vi "thermometric_station.vi"() -> ()   [LabVIEW 2017]
uses:
  dd87deb7-d795-4f28-a263-11bfb0a382d3.vi
  <vilib>/MakerHub/LINX/Public/Utilities/Open Serial.vi
  <vilib>/Utility/file.llb/Write Delimited Spreadsheet (string).vi
  <vilib>/MakerHub/LINX/LMH-LINX.lvlib
panel:
  in  "Stop":bool
  in  "Tab Control":T1(tab)
  out "Value Change":bool
  in  "Acquisition time":string(combo)
  in  "Save Button":bool
  out "Temperature (C)":u8(knob) scale=0.0..50.0
  out "Humidity (%)":u8(knob) scale=0.0..100.0
  in  "Serial Port":refnum<visa-resource-name>="N/A"
  out "Humidity":u8(graph)=43
  out "Temperature":u8(graph)
  out "HTML Content":string
  out "Cleaned Content":string
  out "Error Out":errorcluster
  out "Data":string[](array[string])
  in  "Table":string(combo)
  in  "Connection Information":path
  in  "Columns":string[](array[string])
  in  "Condition":string(combo)
  out "DB read":string[][](array[string])
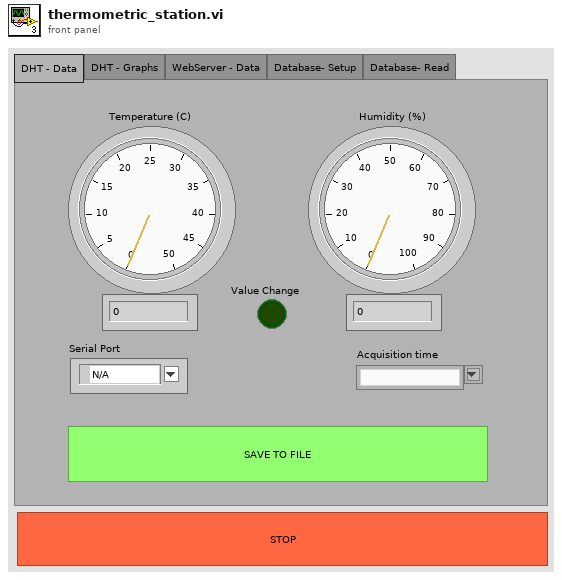
[diagram p1: front panel]
types:
  T1 = enum32{"DHT - Data", "DHT - Graphs", "WebServer - Data", "Database- Setup", "Database- Read"}
  T2 = typedef "LMH-LINX.lvlib/LINX Ref.ctl" = cluster{"IO":T3, "Interface":T4, "LINX Device Config":T5}
  T3 = typedef "LMH-LINX.lvlib/Platform.ctl" = enum16{"Remote", "Local"}
  T4 = typedef "LMH-LINX.lvlib/Interface.ctl" = enum16{"Serial", "TCP"}
  T5 = typedef "LMH-LINX.lvlib/Device.lvlib/LINX Device Config.ctl" = cluster{"Interface":T4, "COM Port":refnum<visa-resource-name>, "TCP Configuration":T6, "Device Family":u8, "Device ID":u8, "Device Name":string, "TCP Ref":refnum<k5>, "Channels":T7}
  T6 = typedef "LMH-LINX.lvlib/Device.lvlib/TCP Config.ctl" = cluster{"IP Address":string, "Port":u16}
  T7 = typedef "LMH-LINX.lvlib/Channels.ctl" = cluster{"DI":u8[], "DO":u8[], "AI":u8[], "AO":u8[], "PWM":u8[], "QE":u8[], "UART":u8[], "I2C 2":u8[], "SPI":u8[], "CAN":u8[], "Servo":u8[], "AI Ref (V)":dbl, "AI Resolution (Bits)":u8, "AO Ref (V)":dbl, "AO Resolution (Bits)":u8}
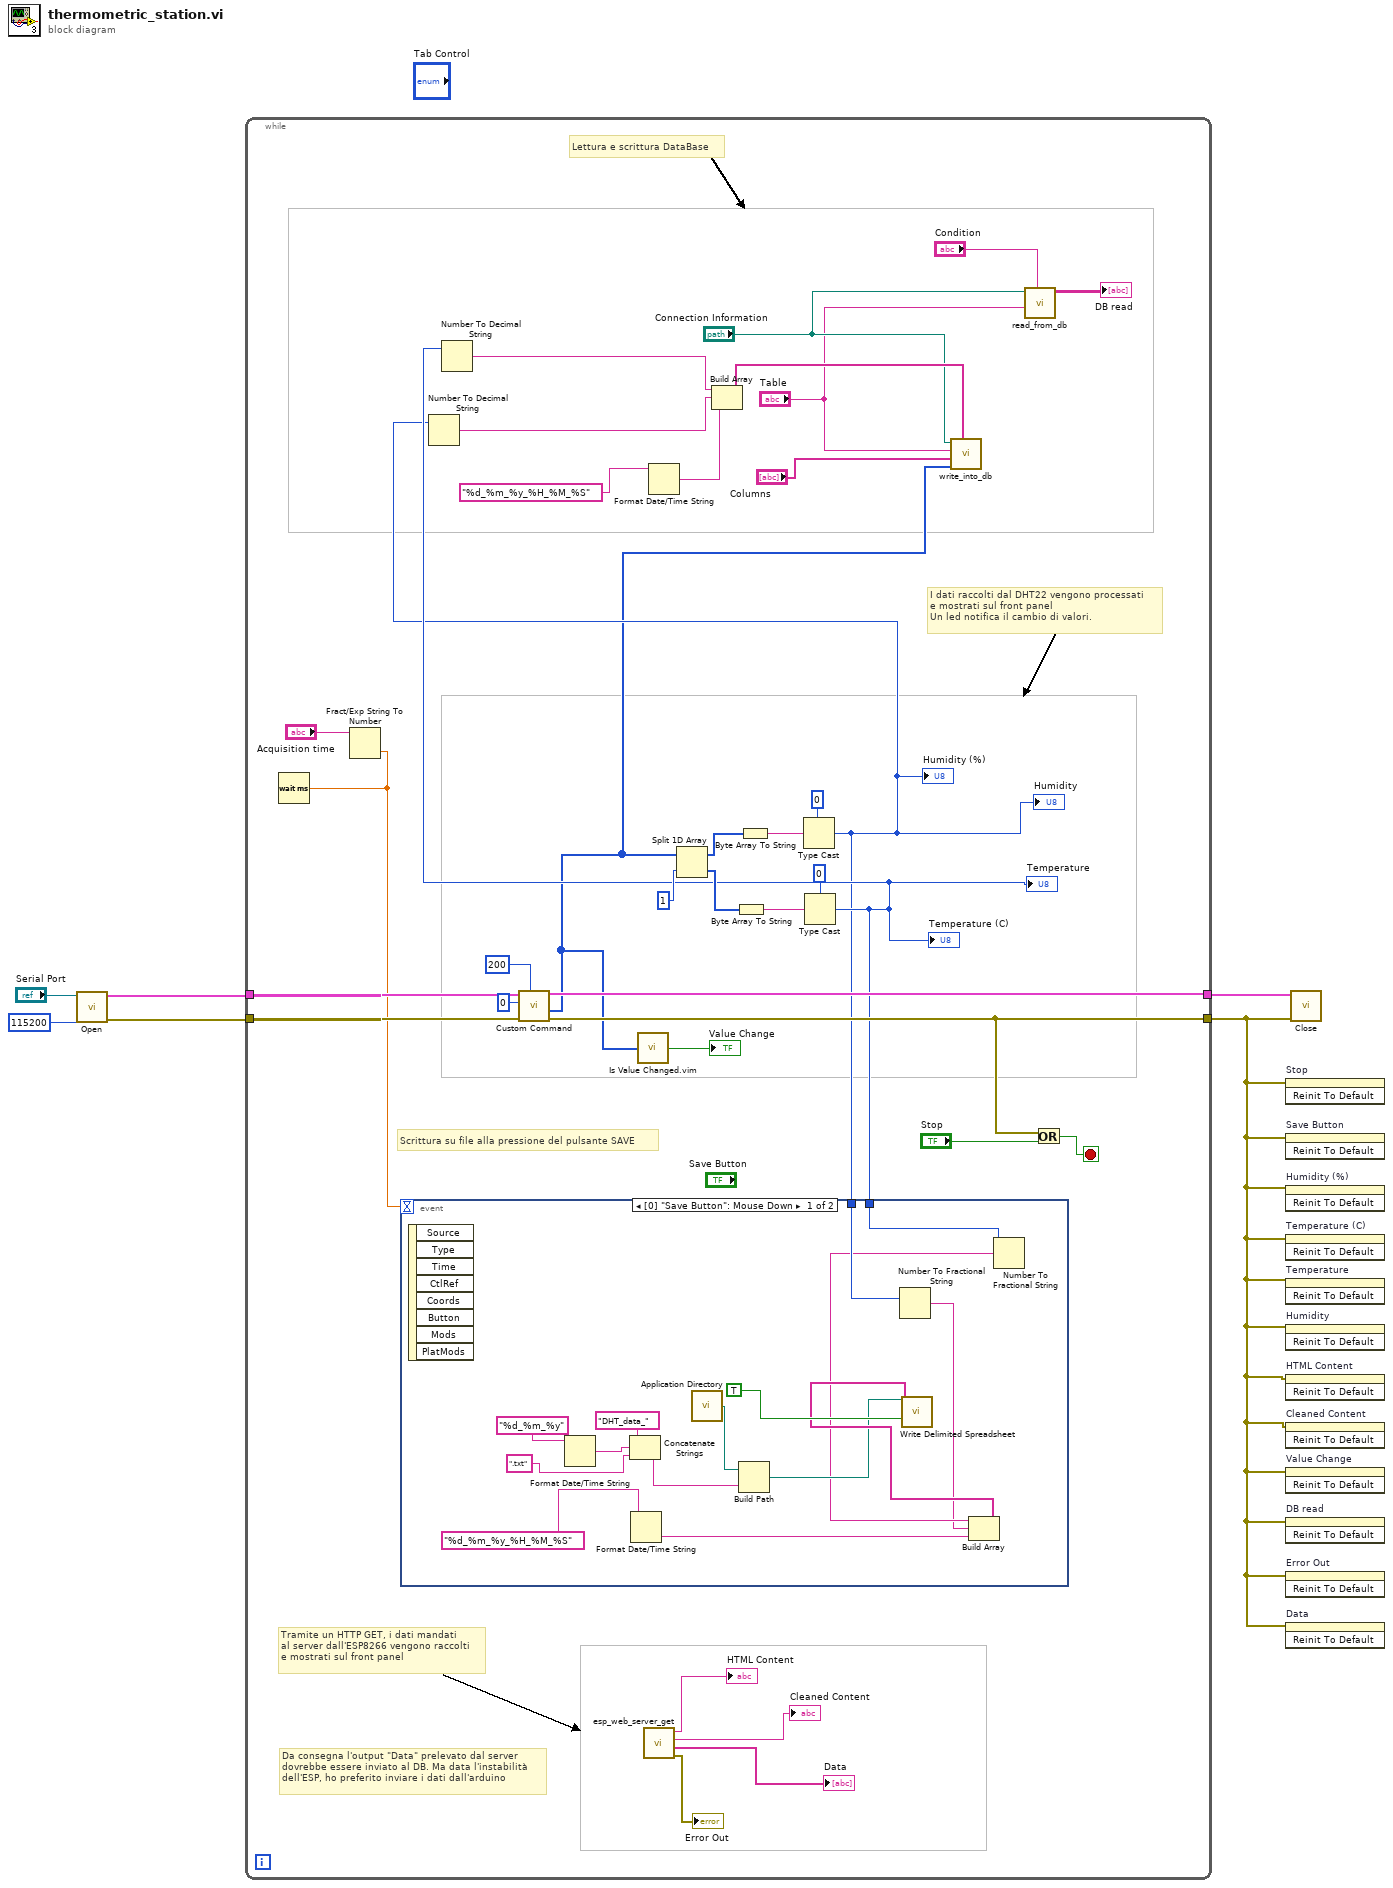
[diagram p0: block diagram]
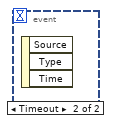
[diagram p2: hidden frame]
diagram:
  n1 = call-poly <vilib>:"Open.vi"("Baud Rate Override"=u32 115200, "Serial Port"="Serial Port") -> ("Error Out"=w5:errorcluster, "LINX Resource"=w6:T2)  [unwired: 7 in, 1 out]
  n2 = while {
    tunnel: w6 -> [w41]
    tunnel: w5 -> [w40]
    tunnel: [w39] -> w4
    tunnel: [w24] -> w1
    stop <- w37 stop-if-true
    # "Da consegna l'output \"Data\" prelevato dal server\ndovrebbe essere inviato al DB. Ma data l'instabilità\ndell'ESP, ho preferito inviare i dati dall'arduino"
    # "Tramite un HTTP GET, i dati mandati\nal server dall'ESP8266 vengono raccolti\ne mostrati sul front panel"
    # "I dati raccolti dal DHT22 vengono processati\ne mostrati sul front panel\nUn led notifica il cambio di valori."
    # "Lettura e scrittura DataBase"
    # "Scrittura su file alla pressione del pulsante SAVE"
    n3 = Fract/Exp String To Number(string="Acquisition time") -> (number=w7:dbl)  [unwired: 3 in, 1 out]
    n4 = Wait (ms)(milliseconds to wait=w7) -> ()  [unwired: 1 out]
    n5 = call <vilib>:"Custom Command.vi"("Timeout (100 ms)"=200, "Error In"=w40, "Custom Command Number"=u16 0, "LINX Resource"=w41) -> ("Error Out"=w24:errorcluster, "Response"=w12:u8[], "LINX Resource"=w39:T2)  [unwired: 4 in, 1 out]
    n6 = call "Is Value Changed.vim"("value"=w12) -> ("changed or first call?"=→"Value Change":bool)
    n7 = call "esp_web_server_get.vi"() -> ("error out"=→"Error Out":errorcluster, "Data"=→"Data":string[], "Cleaned Content"=→"Cleaned Content":string, "HTML Content"=→"HTML Content":string)  [unwired: 8 in]
    n8 = Format Date/Time String(time format string (%c)="%d_%m_%y_%H_%M_%S") -> (date/time string=w18:string)  [unwired: 2 in]
    n9 = Split 1D Array(array=w12, index=1) -> (first subarray=w35:u8[], second subarray=w34:u8[])
    n10 = Byte Array To String(unsigned byte array=w34) -> (string=w29:string)
    n11 = Byte Array To String(unsigned byte array=w35) -> (string=w28:string)
    n12 = Type Cast(type=u8 0, x=w28) -> (*(type *) &x=w22:u8)
    "Humidity (%)" <- w22
    "Humidity" <- w22
    n13 = Number To Decimal String(number=w22) -> (decimal integer string=w20:string)  [unwired: 1 in]
    n14 = Type Cast(type=u8 0, x=w29) -> (*(type *) &x=w23:u8)
    "Temperature (C)" <- w23
    "Temperature" <- w23
    n15 = event shown="[0] \"Save Button\": Mouse Down" {
      selector: _ -> [_ _]
      dyn-events: _ -> [_ _]
      timeout: w7 -> [_ _]
      tunnel: w22 -> [w45 _]
      tunnel: w23 -> [w44 _]
      event "Save Button": Mouse Down {
        n16 = event-data() -> ()  [unwired: 1 in, 8 out]
        n17 = Format Date/Time String(time format string (%c)="%d_%m_%y") -> (date/time string=w50:string)  [unwired: 2 in]
        n18 = Concatenate Strings("DHT_data_", w50, ".txt") -> (w46:string)
        n19 = Format Date/Time String(time format string (%c)="%d_%m_%y_%H_%M_%S") -> (date/time string=w51:string)  [unwired: 2 in]
        n20 = call <vilib>:"Application Directory.vi"() -> ("Application Directory"=w53:path)
        n21 = Build Path(base path=w53, name or relative path=w46) -> (appended path=w52:path)
        n22 = Number To Fractional String(number=w45) -> (F-format string=w42:string)  [unwired: 3 in]
        n23 = Number To Fractional String(number=w44) -> (F-format string=w43:string)  [unwired: 3 in]
        n24 = Build Array(w43, w42, w51) -> (w54:string[])
        n25 = call-poly <vilib>:"Write Delimited Spreadsheet.vi"("file path (dialog if empty)"=w52, "1D data"=w54, "append to file? (new file:F)"=TRUE ("append to file? (F)")) -> ()  [unwired: 11 in, 2 out]
      }
      event Timeout {
        n26 = event-data() -> ()  [unwired: 1 in, 3 out]
      }
    }
    n27 = Number To Decimal String(number=w23) -> (decimal integer string=w21:string)  [unwired: 1 in]
    n28 = Build Array(w21, w20, w18) -> (w25:string[])
    n29 = call "write_into_db.vi"("Array"=w25, "Data"=w12, "Columns"="Columns", "Table"="Table", "connection information"="Connection Information") -> ()  [unwired: 7 in]
    n30 = call "read_from_db.vi"("condition"="Condition", "table"="Table", "connection information"="Connection Information") -> ("data"=→"DB read":string[][])  [unwired: 8 in]
    n31 = Or(x=w24, y="Stop") -> (x .or. y?=w37:bool)
  }
  n32 = invoke on="Stop" class="Bool (strict)" method="Reinit To Default"(error in=w1) -> ()  [unwired: 2 in, 3 out]
  n33 = invoke on="Save Button" class="Bool" method="Reinit To Default"(error in=w1) -> ()  [unwired: 2 in, 3 out]
  n34 = invoke on="Humidity (%)" class="Knob (strict)" method="Reinit To Default"(error in=w1) -> ()  [unwired: 2 in, 3 out]
  n35 = invoke on="Temperature (C)" class="Knob (strict)" method="Reinit To Default"(error in=w1) -> ()  [unwired: 2 in, 3 out]
  n36 = invoke on="Temperature" class="WFChart (strict)" method="Reinit To Default"(error in=w1) -> ()  [unwired: 2 in, 3 out]
  n37 = invoke on="Humidity" class="WFChart (strict)" method="Reinit To Default"(error in=w1) -> ()  [unwired: 2 in, 3 out]
  n38 = invoke on="HTML Content" class="Str" method="Reinit To Default"(error in=w1) -> ()  [unwired: 2 in, 3 out]
  n39 = invoke on="Cleaned Content" class="Str" method="Reinit To Default"(error in=w1) -> ()  [unwired: 2 in, 3 out]
  n40 = invoke on="Value Change" class="Bool (strict)" method="Reinit To Default"(error in=w1) -> ()  [unwired: 2 in, 3 out]
  n41 = invoke on="DB read" class="Arr (strict)" method="Reinit To Default"(error in=w1) -> ()  [unwired: 2 in, 3 out]
  n42 = invoke on="Error Out" class="Clust (strict)" method="Reinit To Default"(error in=w1) -> ()  [unwired: 2 in, 3 out]
  n43 = invoke on="Data" class="Arr (strict)" method="Reinit To Default"(error in=w1) -> ()  [unwired: 2 in, 3 out]
  n44 = call <vilib>:"Close.vi"("Error In"=w1, "LINX Resource"=w4) -> ()  [unwired: 9 in, 1 out]
